vi "FtoCelcius.vi"() -> ()   [LabVIEW 2021]
panel:
  out "C":dbl(slide) scale=0.0..100.0
  in  "F":dbl(slide) scale=0.0..100.0
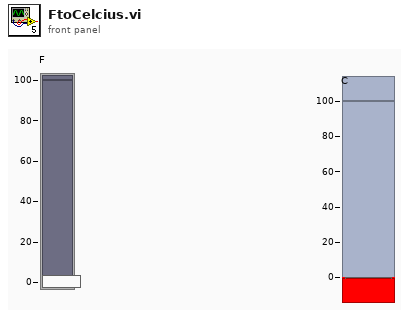
[diagram p1: front panel]
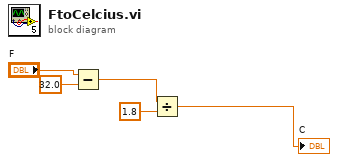
[diagram p0: block diagram]
diagram:
  n1 = Subtract(x="F", y=32.0) -> (x-y=w2:dbl)
  n2 = Divide(x=w2, y=1.8) -> (x/y=→"C":dbl)
